vi "file_cr.vi"(1 "String":string) -> (0 "refnum out":refnum<file>)   [LabVIEW 2015]
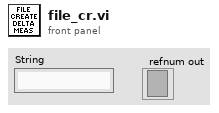
[diagram p1: front panel]
types:
  T1 = enum16{"open", "replace", "create", "open or create", "replace or create", "replace or create with confirmation"}
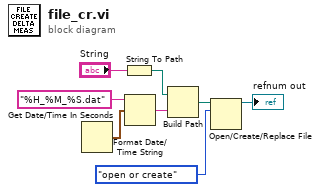
[diagram p0: block diagram]
diagram:
  n1 = Get Date/Time In Seconds() -> (seconds since 1Jan1904=w8:timestamp)
  n2 = String To Path(string="String") -> (path=w2:path)
  n3 = Format Date/Time String(time format string (%c)="%H_%M_%S.dat", seconds (now)=w8) -> (date/time string=w6:string)  [unwired: 1 in]
  n4 = Build Path(base path=w2, name or relative path=w6) -> (appended path=w5:path)
  n5 = Open/Create/Replace File(file path (use dialog)=w5, operation (0:open)=T1."open or create") -> (refnum out=→"refnum out":refnum<file>)  [unwired: 4 in, 2 out]
